vi "搜寻平台起始点.vi"(4 "滤波后数组":dbl[](array[numeric])) -> (1 "stage_start":i32)   [LabVIEW 2011]
doc: "搜索第一个平台的起始点"
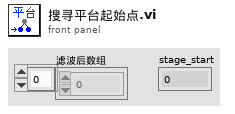
[diagram p1: front panel]
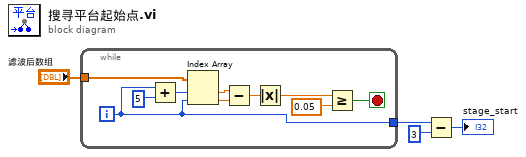
[diagram p0: block diagram]
diagram:
  n1 = while {
    tunnel: "滤波后数组" -> [w14]
    tunnel: [w8] -> w2
    i -> [w8]
    stop <- w6 stop-if-true
    n2 = Add(x=w8, y=5) -> (x+y=w13:i32)
    n3 = Index Array(array=w14, index #1=w13, index #2=w8) -> (element #1=w12:dbl, element #2=w7:dbl)
    n4 = Subtract(x=w12, y=w7) -> (x-y=w11:dbl)
    n5 = Absolute Value(x=w11) -> (abs(x)=w10:dbl)
    n6 = Greater Or Equal?(x=w10, y=0.05) -> (x >= y?=w6:bool)
  }
  n7 = Subtract(x=w2, y=3) -> (x-y=→"stage_start":i32)
